vi "Add Click Zones.vi"(10 "click zones to add":T1[](array[typedef]), 11 "array in":T2) -> (3 "array out":T2)   [LabVIEW 2017, in "NI_Robotics_Configure Steering Frame.lvlib"]
uses:
  <vilib>/robotics/Dialog/Configure Steering Frame/NI_Robotics_Configure Steering Frame.lvlib
  <vilib>/robotics/Dialog/Configure Steering Frame/Click Zone.ctl
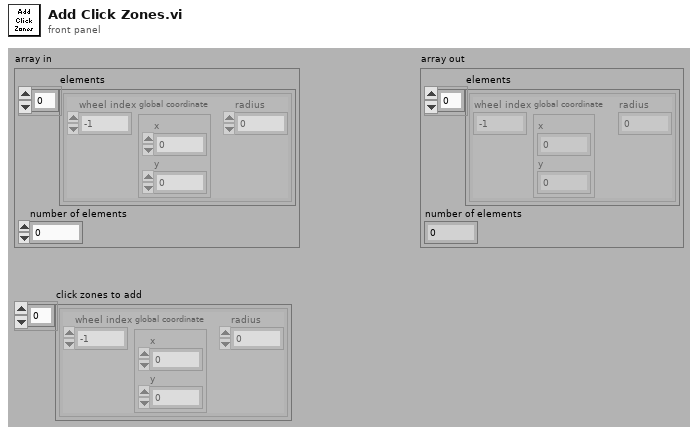
[diagram p1: front panel]
types:
  T1 = typedef "NI_Robotics_Configure Steering Frame.lvlib/Click Zone.ctl" = cluster{"wheel index":i32, "global coordinate":cluster{"x":dbl, "y":dbl}, "radius":dbl}
  T2 = cluster{"elements":T1[], "number of elements":i32}
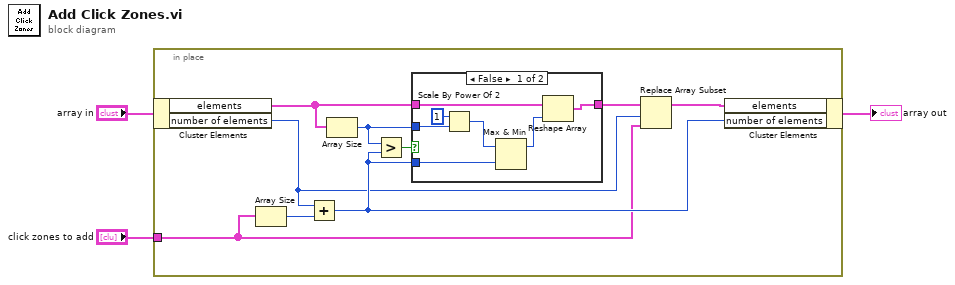
[diagram p0: block diagram]
diagram:
  n1 = in-place {
    in-place-border: "click zones to add" -> [w7]
    n2 = in-place-cluster #1("array in") -> ("elements"=w5:T1[], "number of elements"=w6:i32)
    n3 = Array Size(array=w7) -> (size(s)=w12:i32)
    n4 = Add(x=w6, y=w12) -> (x+y=w10:i32)
    n5 = Array Size(array=w5) -> (size(s)=w4:i32)
    n6 = Greater?(x=w4, y=w10) -> (0:w11:bool)
    n7 = case shown="False" w11 {
      tunnel: w5 -> [w15 w20]
      tunnel: [w13 w20] -> w8
      tunnel: w4 -> [w19 _]
      tunnel: w10 -> [w17 _]
      frame False {
        n8 = Scale By Power Of 2(n=1, x=w19) -> (x*2^n=w16:i32)
        n9 = Max & Min(x=w16, y=w17) -> (max(x,y)=w14:i32)  [unwired: 1 out]
        n10 = Reshape Array(w15, w14) -> (w13:T1[])
      }
      frame True {
      }
    }
    n11 = Replace Array Subset(array=w8, new element=w7, index=w6) -> (w9:T1[])
    n12 = in-place-cluster #1("elements"=w9, "number of elements"=w10) -> (→"array out":T2)
  }
